vi "AskForConnectedCCDsMODIFIED.vi"(7 "DiscoverDevices in":T1, 8 "error in (no error)":errorcluster, 10 "timeout for receiving data [ms]":i32=5000, 11 "Communicator in":refnum<class "Communicator.lvclass">) -> (0 "error out":errorcluster, 2 "DiscoverDevices out":T1, 3 "Communicator out":refnum<class "Communicator.lvclass">)   [LabVIEW 2023, in "DeviceManager.lvlib"]
uses:
  DiscoverDevices (Reply Payload)--cluster.ctl
  Classes/Mono/Monochromator.lvclass
  Classes/CCD/CCD.lvclass
  C:/Users/grju/Desktop/AbgelegteDokumente/Kunden/Horiba/horiba-labview-sdk/Source/Classes/GenericDevice/GenericDevice.lvclass
  Classes/SCD/SCD.lvclass
  Classes/Communicator/Communicator.lvclass
  DeviceManager.lvlib
  Classes/GenericDevice/GenericDevice.lvclass
panel:
  # "Connector Pane"
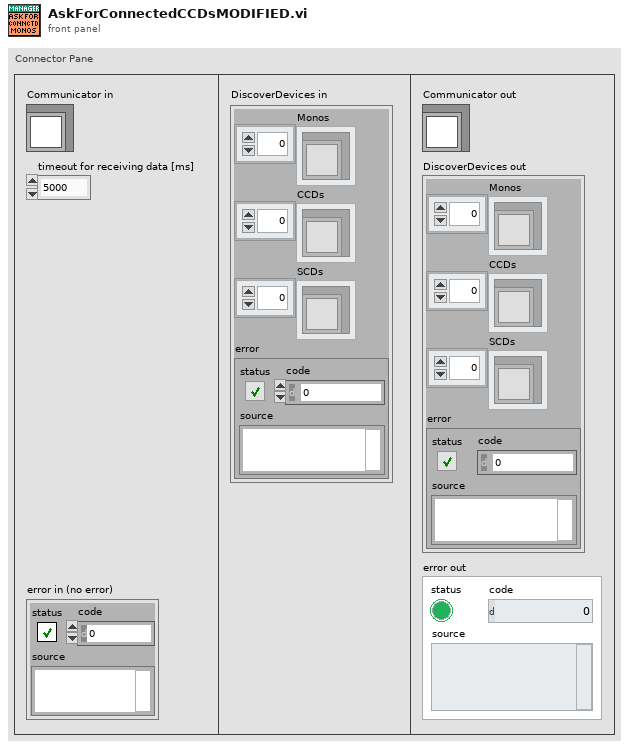
[diagram p1: front panel]
types:
  T1 = typedef "DeviceManager.lvlib/DiscoverDevices (Reply Payload)--cluster.ctl" = cluster{"Monos":refnum<class "Monochromator.lvclass">[], "CCDs":refnum<class "CCD.lvclass">[], "SCDs":refnum<class "SCD.lvclass">[], "error":errorcluster}
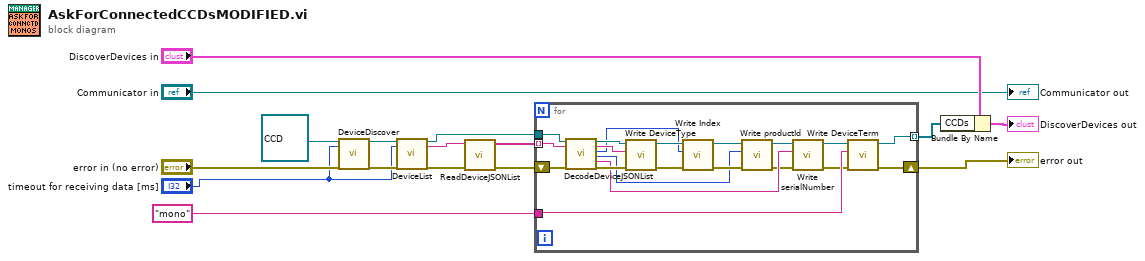
[diagram p0: block diagram]
diagram:
  n1 = call "DeviceDiscover.vi"("GenericDevice in"=refnum<class "CCD.lvclass"> refnum ("CCD.lvclass"), "Delay between send and receive [ms]"="timeout for receiving data [ms]", "error in (no error)"="error in (no error)") -> ("GenericDevice out"=w9:refnum<class "CCD.lvclass">, "error out"=w7:errorcluster)  [unwired: 11 in, 4 out]
  n2 = call "DeviceList.vi"("GenericDevice in"=w9, "Delay between send and receive [ms]"="timeout for receiving data [ms]", "error in (no error)"=w7) -> ("GenericDevice out"=w8:refnum<class "CCD.lvclass">, "results-JSON string"=w3:string, "error out"=w2:errorcluster)  [unwired: 11 in, 3 out]
  n3 = call "ReadDeviceJSONList.vi"("error in"=w2, "JSON"=w3) -> ("error out"=w12:errorcluster, "table of devices"=w13:string[])  [unwired: 8 in]
  n4 = for {
    tunnel: w13 -> [w30] mode=indexing
    shift-right: [w25] -> w14
    shift-left: w12 -> [w28]
    tunnel: w8 -> [w29]
    tunnel: [w26] -> w11 mode=indexing
    tunnel: "mono" -> [w27]
    n5 = call "DecodeDeviceJSONList.vi"("GenericDevice in"=w29, "JSON"=w30, "error in"=w28) -> ("GenericDevice out"=w36:refnum<class "CCD.lvclass">, "deviceType"=w32:string, "index"=w31:i32, "productId"=w17:i32, "serialNumber"=w24:string, "error out"=w34:errorcluster)  [unwired: 10 in, 1 out]
    n6 = call-dynamic "Write DeviceType.vi"("error in (no error)"=w34, "device type"=w32, "CCD in"=w36) -> ("error out"=w33:errorcluster, "CCD out"=w35:refnum<class "CCD.lvclass">)  [unwired: 7 in]
    n7 = call-dynamic "Write Index.vi"("error in (no error)"=w33, "Index"=w31, "CCD in"=w35) -> ("error out"=w21:errorcluster, "CCD out"=w23:refnum<class "CCD.lvclass">)  [unwired: 7 in]
    n8 = call-dynamic "Write productId.vi"("error in (no error)"=w21, "productId"=w17, "CCD in"=w23) -> ("error out"=w20:errorcluster, "CCD out"=w22:refnum<class "CCD.lvclass">)  [unwired: 7 in]
    n9 = call-dynamic "Write serialNumber.vi"("error in (no error)"=w20, "serialNumber"=w24, "CCD in"=w22) -> ("error out"=w18:errorcluster, "CCD out"=w19:refnum<class "CCD.lvclass">)  [unwired: 7 in]
    n10 = call-dynamic "Write DeviceTerm.vi"("error in (no error)"=w18, "deviceTerm"=w27, "CCD in"=w19) -> ("error out"=w25:errorcluster, "CCD out"=w26:refnum<class "CCD.lvclass">)  [unwired: 7 in]
  }
  "error out" <- w14
  n11 = Bundle By Name(cluster="DiscoverDevices in", "CCDs"=w11) -> (→"DiscoverDevices out":T1)
  "Communicator out" <- "Communicator in"
